vi "GF_CodeTimer.vi"(0 "error in":errorcluster) -> (1 "Time":u32, 2 "error out":errorcluster)   [LabVIEW 2009]
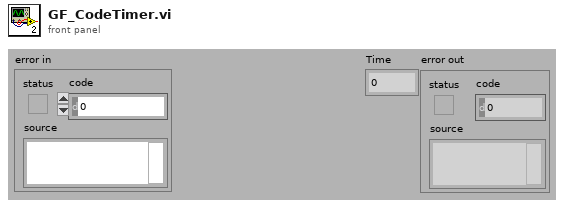
[diagram p1: front panel]
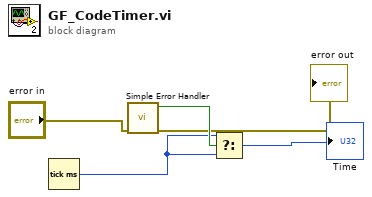
[diagram p0: block diagram]
diagram:
  n1 = Tick Count (ms)() -> (millisecond timer value=w3:u32)
  n2 = call <vilib>:"Simple Error Handler.vi"("error in (no error)"="error in") -> ("error?"=w4:bool, "error out"=→"error out":errorcluster)  [unwired: 4 in, 3 out]
  n3 = Select(t=w3, s=w4, f=w3) -> (s? t:f=→"Time":u32)
